vi "Acquisition Message Loop.vi"(8 "error in (no error)":errorcluster, 11 "Message Queues in":T1) -> (0 "error out":errorcluster)   [LabVIEW 2016, in "Acquisition.lvlib"]
uses:
  Acquisition.lvlib
  Support VIs/Message Queue/Message Queues.ctl
  Support VIs/Message Queue/Message.ctl
  <vilib>/Utility/error.llb/Error Cluster From Error Code.vi
  <vilib>/ErrorRing/Error Ring.xnode
  Support VIs/Message Queue/Message Queue.lvlib
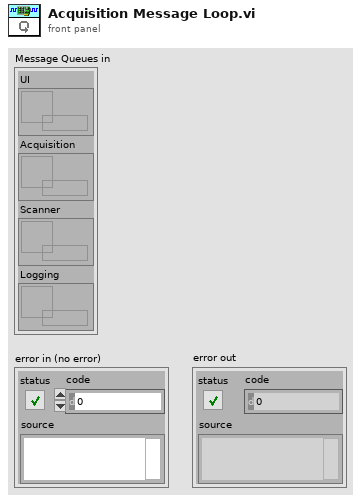
[diagram p1: front panel]
types:
  T1 = typedef "Message Queue.lvlib/Message Queues.ctl" = cluster{"UI":refnum<queue>, "Acquisition":refnum<queue>, "Scanner":refnum<queue>, "Logging":refnum<queue>}
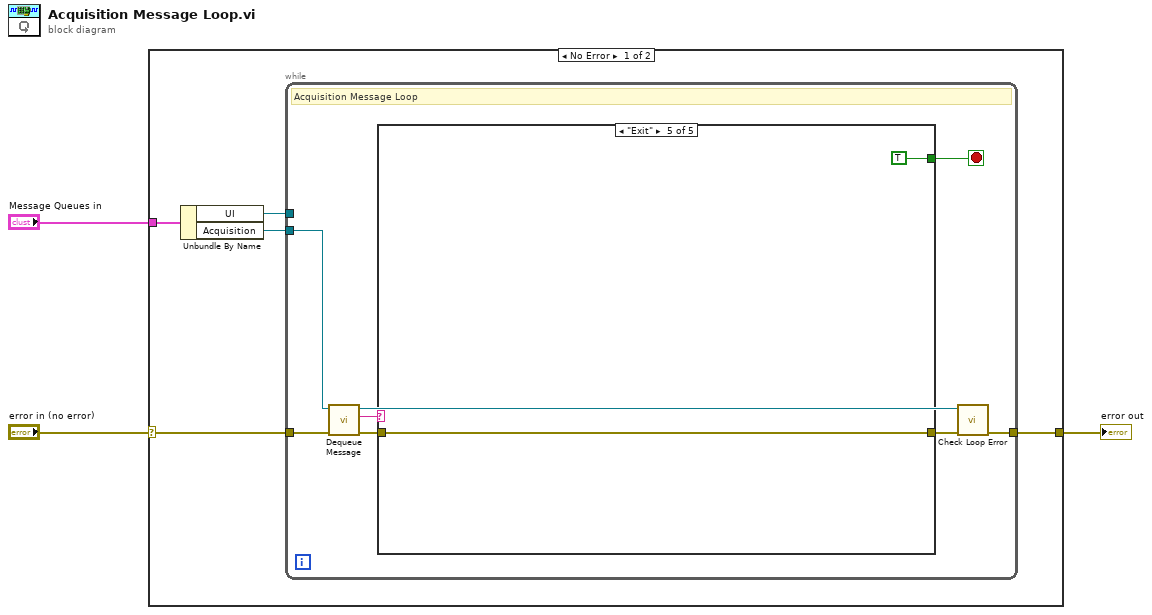
[diagram p0: block diagram]
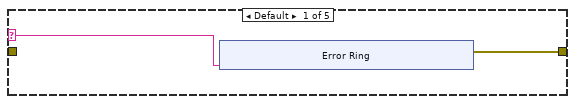
[diagram p2: hidden frame]
diagram:
  n1 = case shown="No Error" "error in (no error)" {
    selector: "error in (no error)" -> [w8 w31]
    tunnel: "Message Queues in" -> [w6 _]
    tunnel: [w7 w31] -> w1
    frame No Error {
      n2 = Unbundle By Name(w6) -> ("UI"=w5:refnum<queue>, "Acquisition"=w4:refnum<queue>)
      n3 = while {
        tunnel: w8 -> [w15]
        tunnel: [w11] -> w7
        tunnel: w5 -> [_]
        tunnel: w4 -> [w16]
        stop <- w9 stop-if-true
        # "Acquisition Message Loop"
        n4 = call "Dequeue Message.vi"("error in (no error)"=w15, "Message Queue in"=w16) -> ("error out"=w13:errorcluster, "State"=w14:string, "Message Queue out"=w10:refnum<queue>)  [unwired: 6 in, 1 out]
        n5 = case shown="\"Exit\"" w14 {
          selector: w14 -> [w17 _ _ _ _]
          tunnel: w13 -> [_ w26 w27 w28 w30]
          tunnel: [w18 w26 w27 w28 w30] -> w12
          tunnel: [_ _ _ _ TRUE] -> w9
          frame Default {
            n6 = xnode "Error Ring"("parameter 0"=w17) -> ("error out"=w18:errorcluster)
          }
          frame "Initialize" {
          }
          frame "--- MISC ---" {
          }
          frame "Error" {
          }
          frame "Exit" {
          }
        }
        n7 = call "Check Loop Error.vi"("error in (no error)"=w12, "Message Queue in"=w10) -> ("error out"=w11:errorcluster)  [unwired: 7 in, 2 out]
      }
    }
    frame Error {
    }
  }
  "error out" <- w1
